vi "Read Tag.vi"(11 "Abs_Type in":refnum<class "Abs_Type.lvclass">) -> (2 "Tag":string, 3 "Abs_Type out":refnum<class "Abs_Type.lvclass">)   [LabVIEW 2021, in "Abs_Type.lvclass"]
uses:
  Abs_Type.lvclass
  Abs_Type.lvclass/Abs_Type.ctl
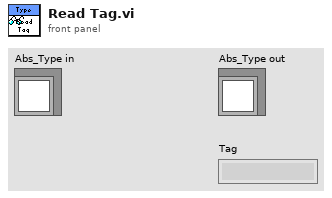
[diagram p1: front panel]
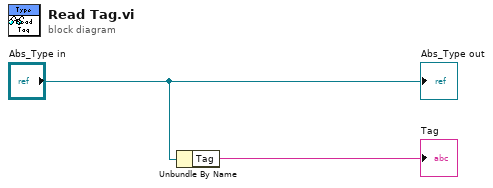
[diagram p0: block diagram]
diagram:
  n1 = Unbundle By Name("Abs_Type in") -> ("Tag"=→"Tag":string)
  "Abs_Type out" <- "Abs_Type in"
